vi "AO Continuous Config Pane.vi"(6 "_SubPanelMessages":refnum<notifier>, 9 "_myEmbeddedToFrameEvent":T7, 10 "_myEmbedded.Exit":refnum<user-event>, 11 "-Property Bundle":cluster{"Name":string, "Value":variant}[](array[cluster])) -> (1 "_Connection Informations":T3, 2 "_Scripter Input":T9)   [LabVIEW 2021]
doc: "Writes values to one or more analog output channels. Use this Express VI to write one or multiple samples for each channel at one time."
uses:
  <vilib>/myRIO/Common/Express VI Framework/xctls/myRIO Channel List/myRIO Channel List.xctl
  <vilib>/myRIO/Common/Express VI Framework/typedefs/Config Pane to Framework Ref.ctl
  <vilib>/myRIO/Common/Express VI Framework/typedefs/Data Validate Ref.ctl
  <vilib>/myRIO/Common/Express VI Framework/typedefs/Scripter Input.ctl
  <vilib>/myRIO/Common/Express VI Framework/typedefs/WireThrough Terminal Names.ctl
  <vilib>/myRIO/Common/Express VI Framework/typedefs/Instrument Driver Method Descriptor Array.ctl
  <vilib>/myRIO/Common/Express VI Framework/typedefs/Instrument Driver Method Descriptor.ctl
  <vilib>/myRIO/Common/Express VI Framework/typedefs/Sub Panel Messages.ctl
  <vilib>/myRIO/Common/Express VI Framework/typedefs/Connection Informations.ctl
  <vilib>/myRIO/Common/Instrument Driver Framework/Utilities/typedefs/Channel Types.ctl
  <vilib>/myRIO/Common/Express VI Framework/vis/Express VI Framework Strings Global.vi
panel:
  in  "Timeout":i32=-1 caption="Timeout:"
  in  "Sample Rate Unit":string="kHz"
  out "_learnMoreLatency":string="No gap exists during continuous generation. Learn more"
  out "_learnMoreFrequency":string="Detailed information about valid update rates for this Express VI. Learn more"
  in  "Wait Until Done?":bool caption="Wait until done?"
  in  "_Validate":bool
  in  "Sample Rate:":dbl=1.0 caption="Update rate:"
  in  "Name:":string="Analog output (continuous)" caption="Node name:"
  in  "Selected Channel List":T1[](xcontrol)=[{"Channel Name"=0, "Channel Alias"="", "Remove Channel"=FALSE, "Index"=0}]
  in  "_Default Alias String":string
  in  "_VI Default Name (Edit and make value default)":string="Analog output (continuous)"
  in  "_WireThrough Info (Edit and make value default)":T4={"WireThrough Top In"="AO (Continuous) Ref In", "WireThrough Bottom In"="error in (no error)", "WireThrough Top Out"="AO (Continuous) Ref Out", "WireThrough Bottom Out"="error out"}
  in  "_Template Array (Edit and make value default)":T5=[{"Function Name"="AO Continuous Smart Write", "VI Path"=path "<vilib>/myRIO/Instrument Drivers/Onboard IO/AO Continuous/vis", "Script"=TRUE, "Inputs"=[{"name"="Channel Names", "value"=variant, "Config Pane Only"=TRUE, "Build Array"=FALSE, "Bundle Cluster"=FALSE, "Show Term"=FALSE, "alias"=[], "Required Input"=FALSE}, {"name"="Sample Rate", "value"=variant, "Config Pane Only"=TRUE, "Build Array"=FALSE, "Bundle Cluster"=FALSE, "Show Term"=FALSE, "alias"=[], "Required Input"=FALSE}, {"name"="Data To Write", "value"=variant, "Config Pane Only"=FALSE, "Build Array"=TRUE, "Bundle Cluster"=FALSE, "Show Term"=TRUE, "alias"=[], "Required Input"=TRUE}, {"name"="Timeout", "value"=variant, "Config Pane Only"=TRUE, "Build Array"=FALSE, "Bundle Cluster"=FALSE, "Show Term"=FALSE, "alias"=[], "Required Input"=FALSE}, {"name"="Wait Until Done?", "value"=variant, "Config Pane Only"=TRUE, "Build Array"=FALSE, "Bundle Cluster"=FALSE, "Show Term"=FALSE, "alias"=[], "Required Input"=FALSE}, {"name"="Stop?", "value"=variant, "Config Pane Only"=FALSE, "Build Array"=FALSE, "Bundle Cluster"=FALSE, "Show Term"=TRUE, "alias"=[], "Required Input"=TRUE}], "Outputs"=[], "VI Class"=enum."Open", "Controls Refs[]"=[], "Inline"=TRUE}]
  in  "_Test Close":bool
  # "User Visible Area"
  # "NOTE: Tab Order has been set\nfor this Front Panel.\n1. Name: (string control)\n2. Add Channel (button)\n3. Selected Channel List (array)\n\nAll other controls are excluded \nfrom Tabbing order\n\nTo exlude a control from context\nhelp prefix its label text with a '-'"
  # "kS/s"
  # "ms"
  # "When you set Stop? terminal to TRUE, this Express VI waits until the write operation completes."
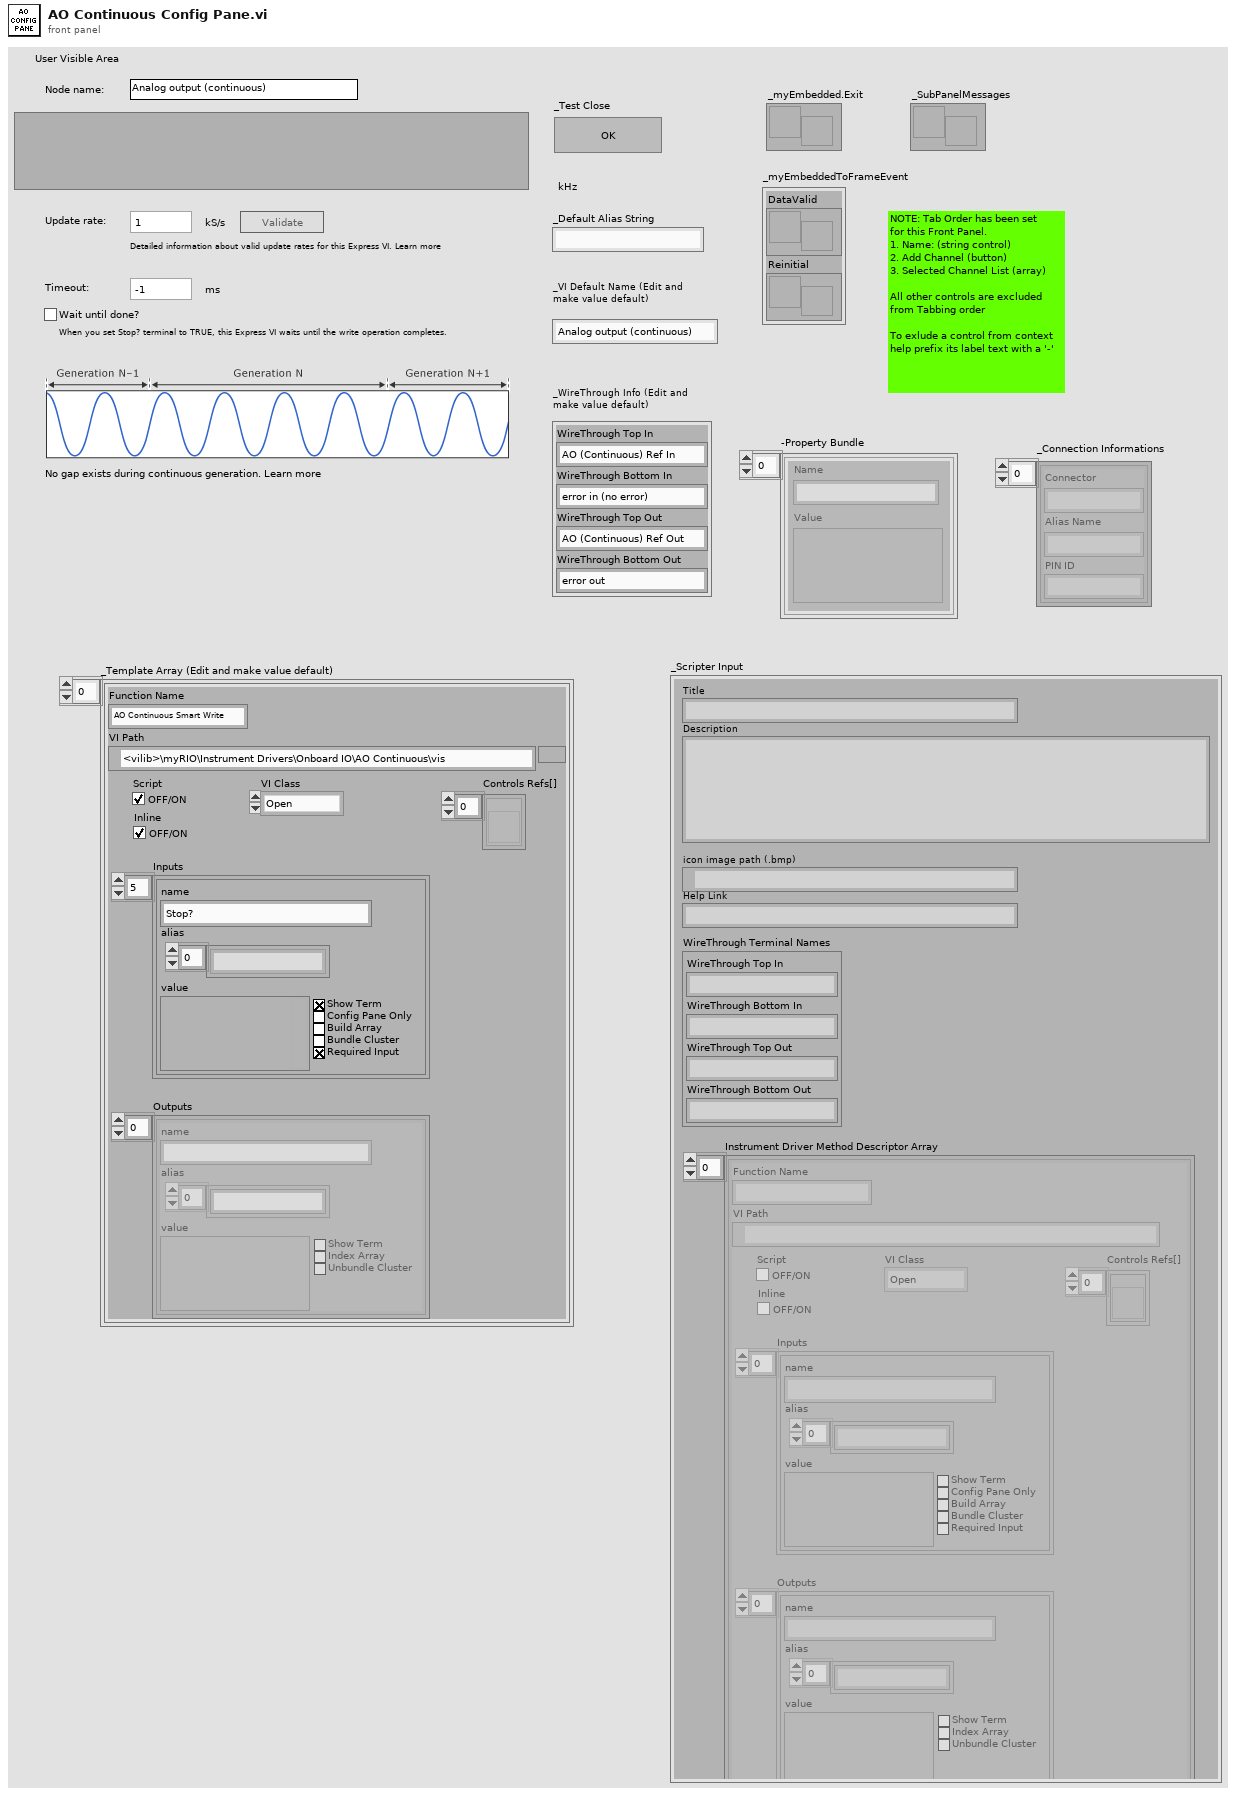
[diagram p1: front panel]
types:
  T1 = typedef "myRIO Channel List.xctl/Channel Data.ctl" = cluster{"Channel Name":u16, "Channel Alias":string, "Remove Channel":T2, "Index":i32}
  T2 = typedef "myRIO Channel List.xctl/Remove Channel.ctl" = bool
  T3 = typedef "Connection Informations.ctl" = cluster{"Connector":string, "Alias Name":string, "PIN ID":string}[]
  T4 = typedef "WireThrough Terminal Names.ctl" = cluster{"WireThrough Top In":string, "WireThrough Bottom In":string, "WireThrough Top Out":string, "WireThrough Bottom Out":string}
  T5 = typedef "Instrument Driver Method Descriptor Array.ctl" = T6[]
  T6 = typedef "Instrument Driver Method Descriptor.ctl" = cluster{"Function Name":string, "VI Path":path, "Script":bool, "Inputs":cluster{"name":string, "value":variant, "Config Pane Only":bool, "Build Array":bool, "Bundle Cluster":bool, "Show Term":bool, "alias":string[], "Required Input":bool}[], "Outputs":cluster{"name":string, "value":variant, "Show Term":bool, "Index Array":bool, "Unbundle Cluster":bool, "alias":string[]}[], "VI Class":enum16{"Open", "Configure", "Data", "Manage", "Close"}, "Controls Refs[]":refnum<vi>[], "Inline":bool}
  T7 = typedef "Config Pane to Framework Ref.ctl" = cluster{"DataValid":T8, "Reinitial":refnum<user-event>}
  T8 = typedef "Data Validate Ref.ctl" = refnum<user-event>
  T9 = typedef "Scripter Input.ctl" = cluster{"Title":string, "Description":string, "icon image path (.bmp)":path, "Help Link":string, "WireThrough Terminal Names":T4, "Instrument Driver Method Descriptor Array":T5}
  T10 = typedef "Channel Types.ctl" = enum32{"Unknown", "AI", "AO", "DIO - DI", "DIO", "DIO - DO", "I2C", "PWM", "Encoder", "SPI", "UART", "Accelerometer", "DIO - LED", "DIO - Button", "AI (N Samples)", "AudioIn (N Samples)", "AO (N Samples)", "AudioOut (N Samples)", "DI (N Samples)", "DO (N Samples)", "AI IRQ", "DI IRQ", "Timer IRQ", "RSL", "Relay", "CAN", "AI (Continuous)", "AO (Continuous)"}
  T11 = typedef "Channel Info.ctl" = cluster{"Channel Name":string, "Alias":string, "Used?":bool, "Not Support?":bool, "Property Bundle":cluster{"Name":string, "Value":variant}[]}
  T12 = typedef "Sub Panel Messages.ctl" = enum16{"Initialized"}
  T13 = enum8{"Enabled", "Disabled", "Disabled and Grayed Out"}
  T14 = cluster{"Connector":string, "Alias Name":string, "PIN ID":string}[]
  T15 = cluster{"name":string, "value":variant, "Config Pane Only":bool, "Build Array":bool, "Bundle Cluster":bool, "Show Term":bool, "alias":string[], "Required Input":bool}[]
  T16 = cluster{"name":string, "value":variant, "Config Pane Only":bool, "Build Array":bool, "Bundle Cluster":bool, "Show Term":bool, "alias":string[], "Required Input":bool}
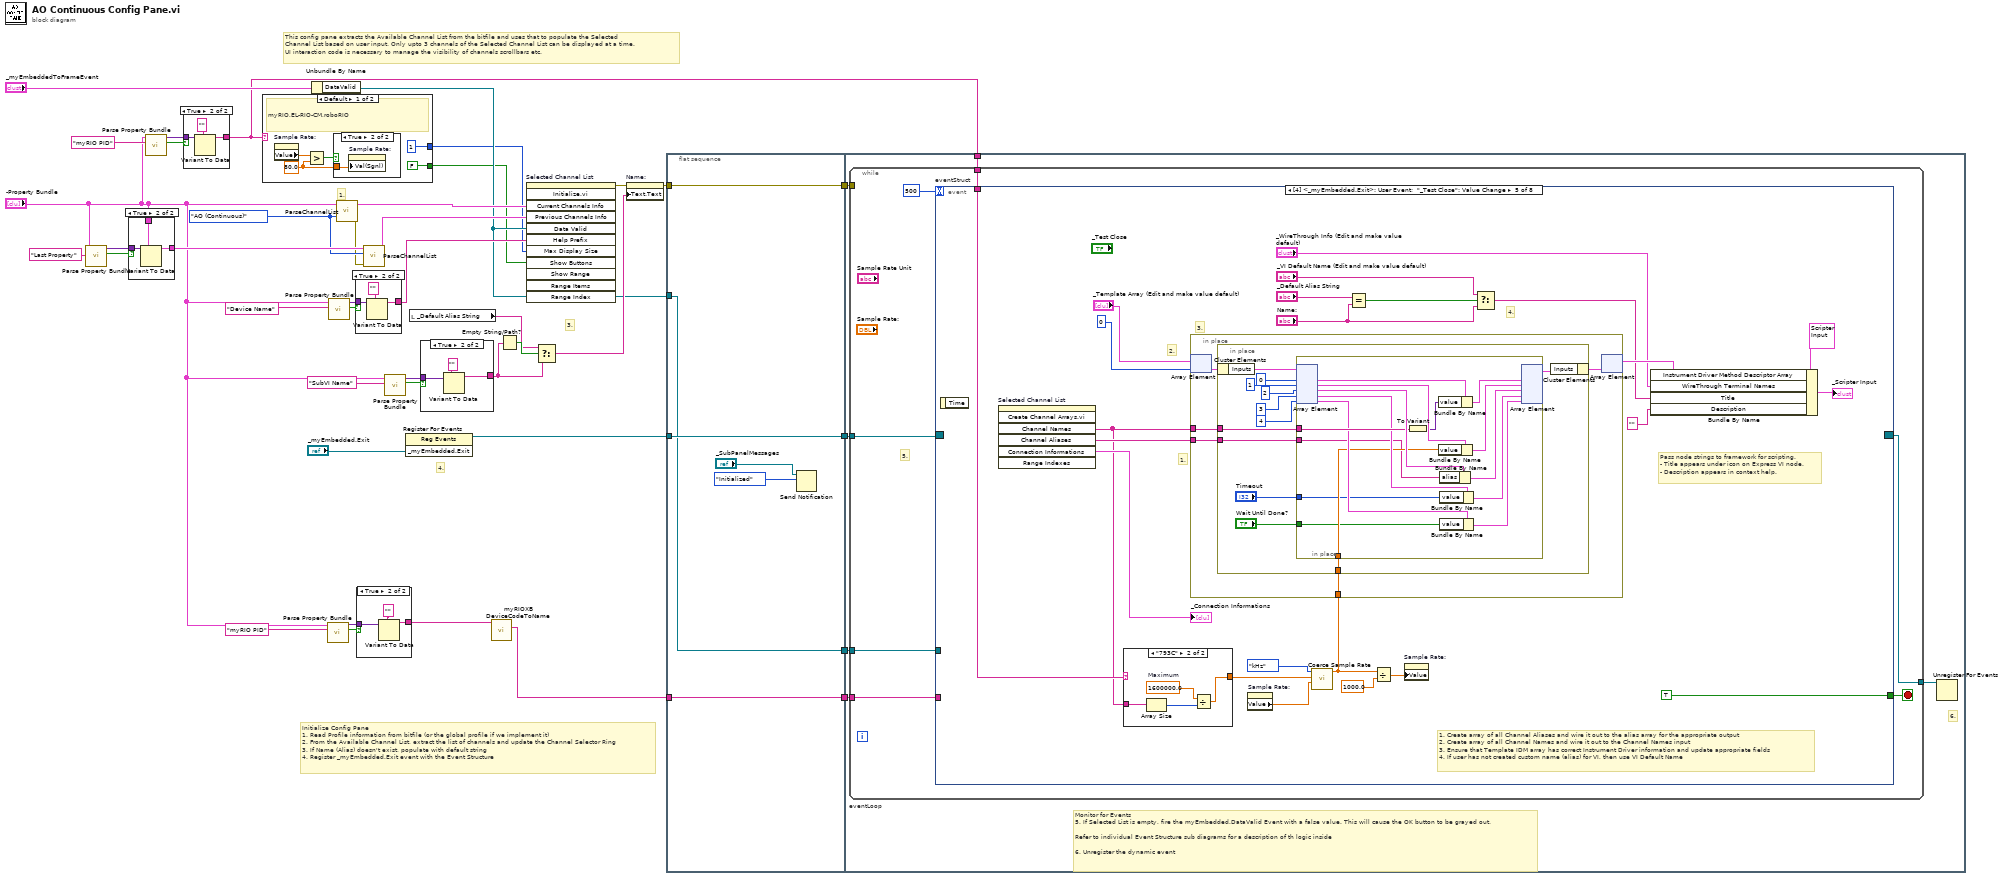
[diagram p0: block diagram]
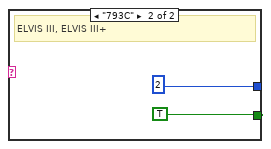
[diagram p3: hidden frame]
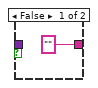
[diagram p4: hidden frame]
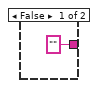
[diagram p5: hidden frame]
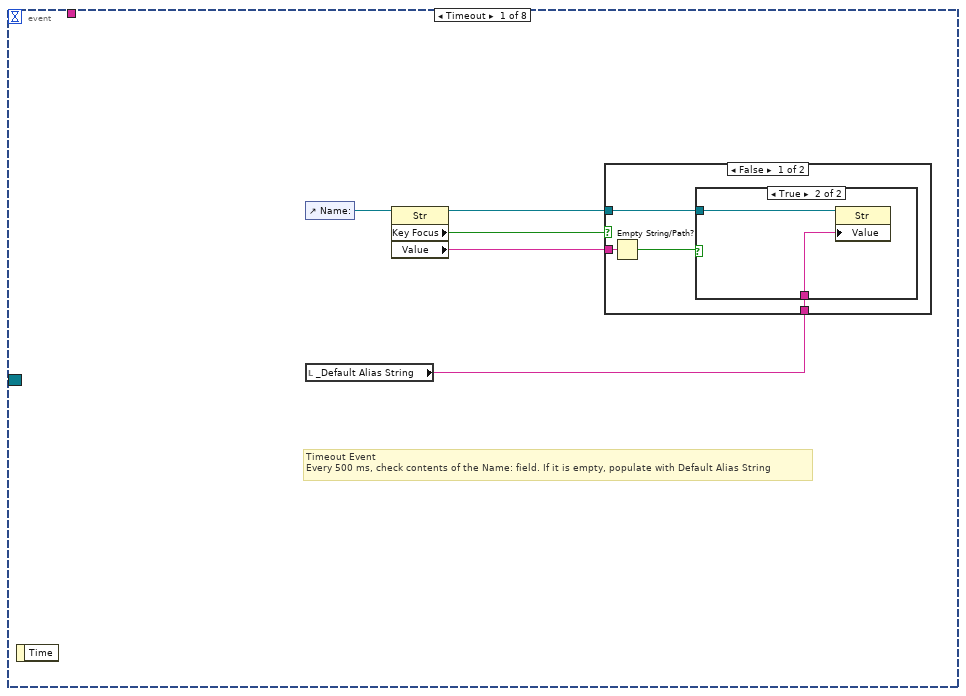
[diagram p6: hidden frame]
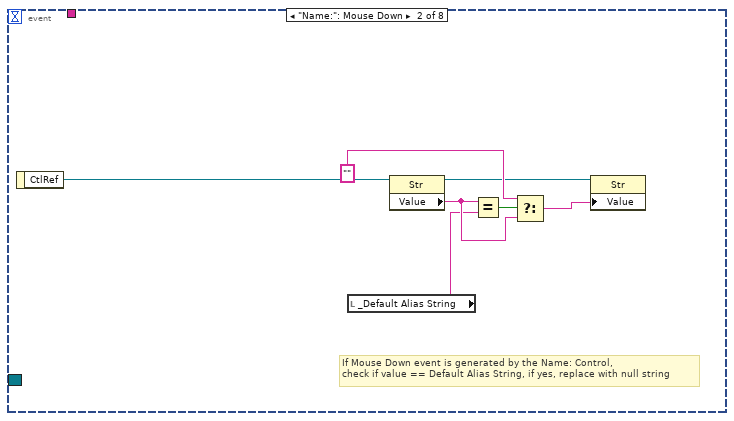
[diagram p9: hidden frame]
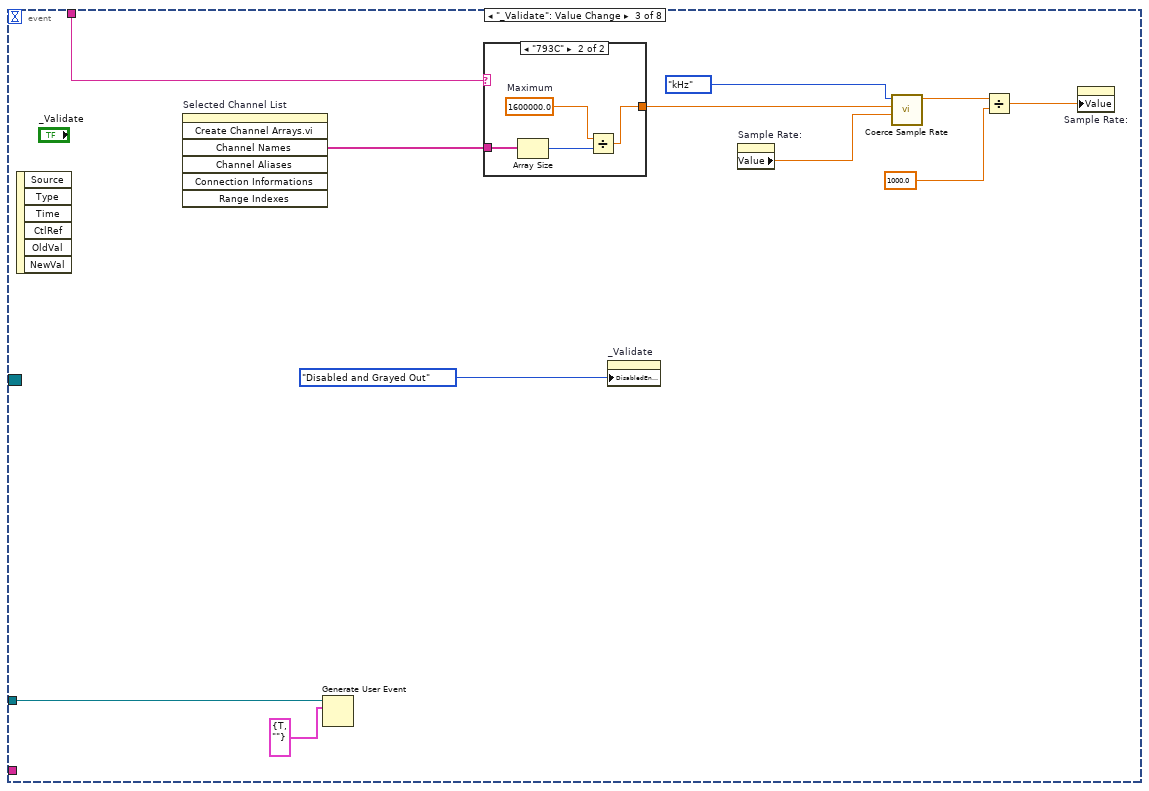
[diagram p10: hidden frame]
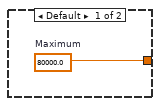
[diagram p11: hidden frame]
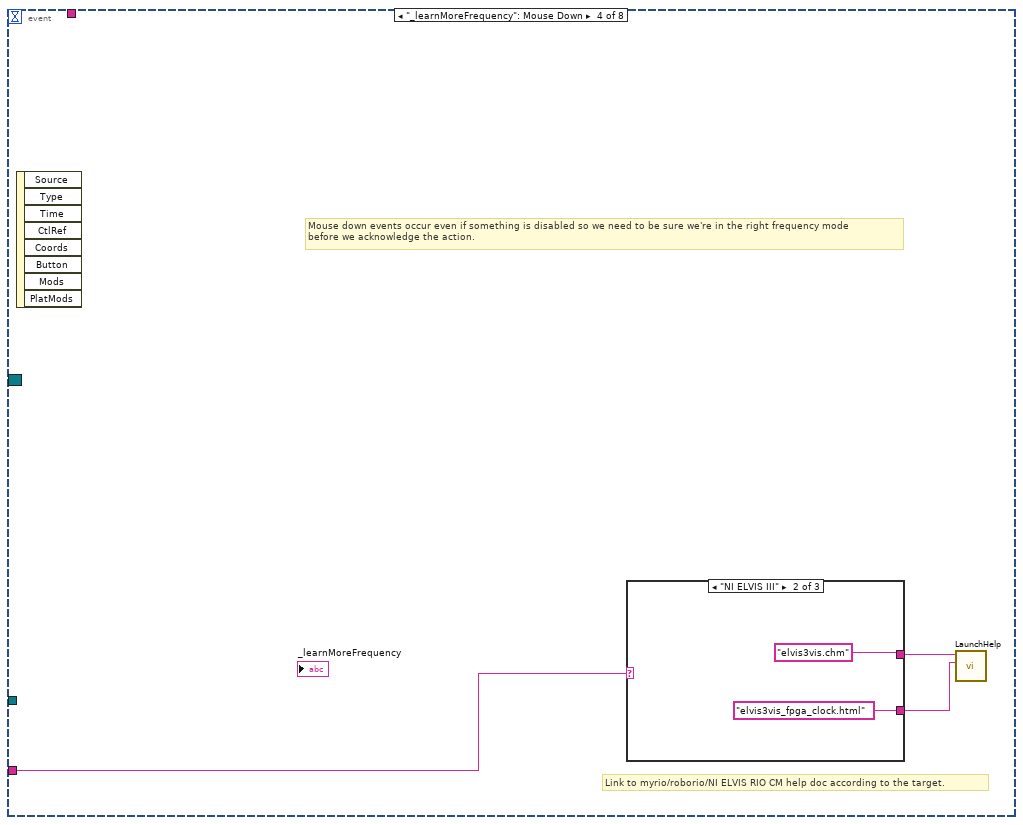
[diagram p12: hidden frame]
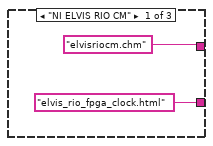
[diagram p13: hidden frame]
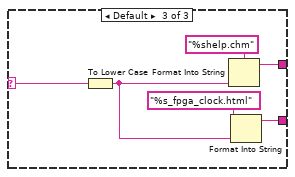
[diagram p14: hidden frame]
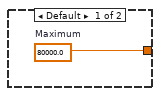
[diagram p15: hidden frame]
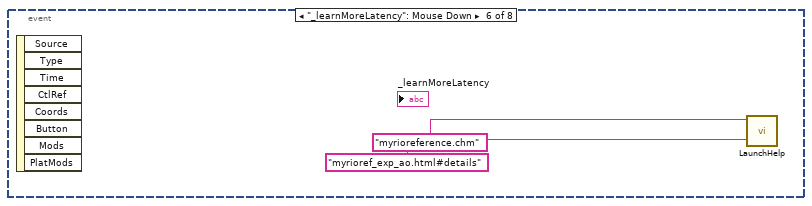
[diagram p16: hidden frame]
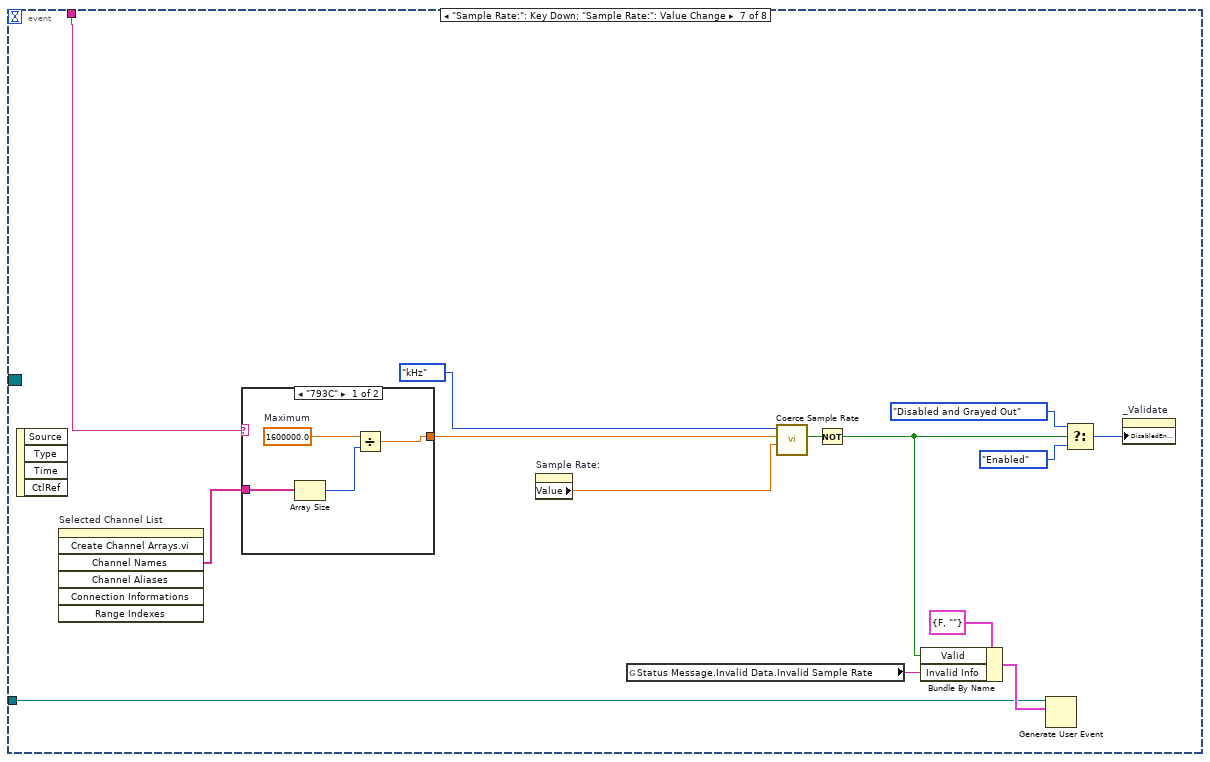
[diagram p17: hidden frame]
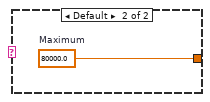
[diagram p18: hidden frame]
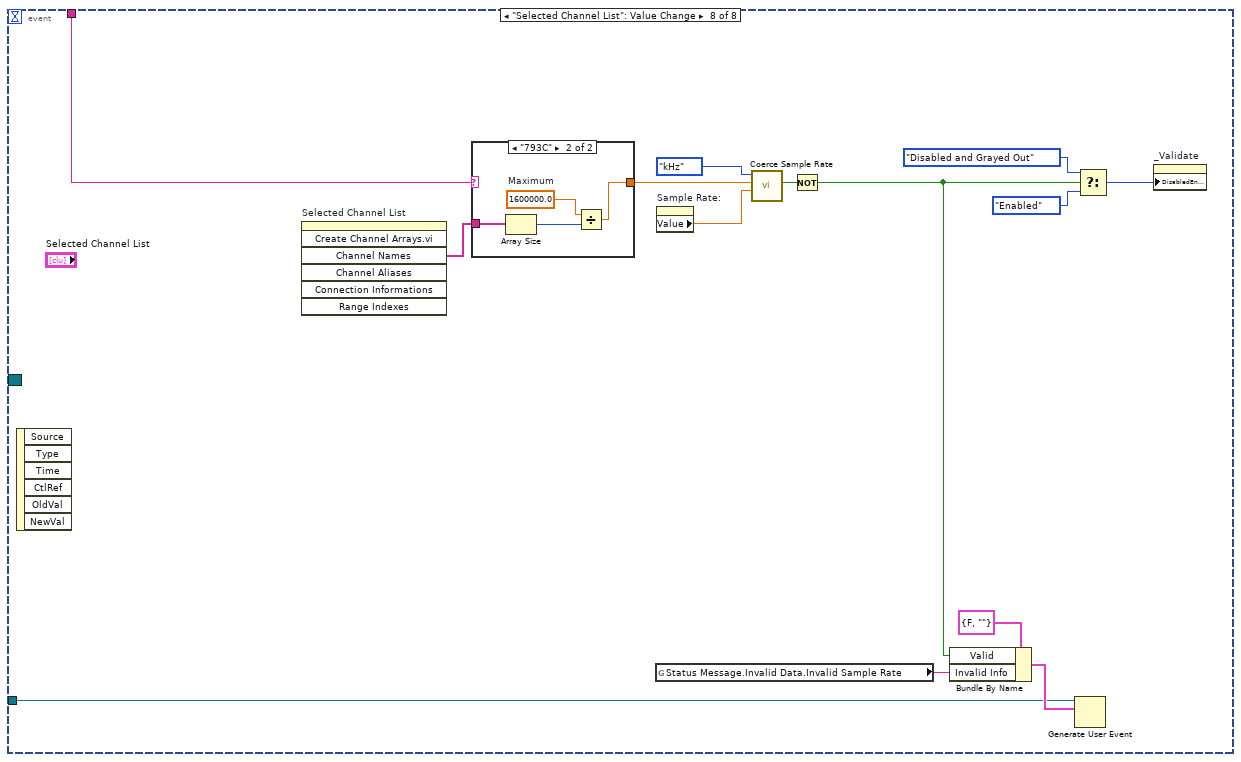
[diagram p19: hidden frame]
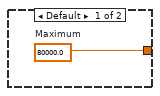
[diagram p20: hidden frame]
diagram:
  w25 = Channel_Types."AO (Continuous)" ("Channel to Read")
  # "3."
  # "1."
  # "This config pane extracts the Available Channel List from the bitfile and uses that to populate the Selected \nChannel List based on user input. Only upto 3 channels of the Selected Channel List can be displayed at a time. \nUI interaction code is necessary to manage the visibility of channels scrollbars etc."
  # "4."
  # "Initialize Config Pane\n1. Read Profile information from bitfile (or the global profile if we implement it)\n2. From the Available Channel List, extract the list of channels and update the Channel Selector Ring\n3. If Name (Alias) doesn't exist, populate with default string\n4. Register _myEmbedded.Exit event with the Event Structure"
  n1 = call <vilib>:"Parse Property Bundle.vi"("Name"="Last Property", "Property Bundle"="-Property Bundle") -> ("Found?"=w27:bool, "Value"=w28:variant)  [unwired: 8 in]
  n2 = case shown="True" w27 {
    tunnel: w28 -> [_ w44]
    tunnel: [_ w43] -> w26
    tunnel: "-Property Bundle" -> [_ w42]
    frame False {
    }
    frame True {
      n3 = Variant To Data(type=w42, Variant=w44) -> (data=w43:cluster{"Name":string, "Value":variant}[])  [unwired: 1 in, 1 out]
    }
  }
  n4 = call <vilib>:"Parse Property Bundle.vi"("Name"="myRIO PID", "Property Bundle"="-Property Bundle") -> ("Found?"=w4:bool, "Value"=w5:variant)  [unwired: 8 in]
  n5 = case shown="True" w4 {
    tunnel: w5 -> [_ w48]
    tunnel: ["" ("Name") w47] -> w1
    frame False {
    }
    frame True {
      n6 = Variant To Data(type="" ("Name"), Variant=w48) -> (data=w47:string)  [unwired: 1 in, 1 out]
    }
  }
  n7 = case shown="Default" w1 {
    tunnel: [FALSE TRUE] -> w3
    tunnel: [1 ("Max Display Size") 2 ("Max Display Size")] -> w2
    frame Default {
      w49 = 80.0 ("y")
      # "myRIO,EL-RIO-CM,roboRIO"
      n8 = property on="Sample Rate:" class="DigNum (strict)"() -> ("Value"=w51:dbl)  [unwired: 2 in, 2 out]
      n9 = Greater?(x=w51, y=w49) -> (0:w50:bool)
      n10 = case shown="True" w50 {
        tunnel: w49 -> [_ w54]
        frame False {
        }
        frame True {
          n11 = property on="Sample Rate:" class="DigNum (strict)"("Val(Sgnl)"=w54) -> ()  [unwired: 2 in, 2 out]
        }
      }
    }
    frame "793C" {
      # "ELVIS III, ELVIS III+"
    }
  }
  n12 = Unbundle By Name("_myEmbeddedToFrameEvent") -> ("DataValid"=w15:T8)
  n13 = call <vilib>:"Parse Property Bundle.vi"("Name"="myRIO PID", "Property Bundle"="-Property Bundle") -> ("Found?"=w11:bool, "Value"=w12:variant)  [unwired: 8 in]
  n14 = call <vilib>:"Parse Property Bundle.vi"("Name"="Device Name", "Property Bundle"="-Property Bundle") -> ("Found?"=w21:bool, "Value"=w20:variant)  [unwired: 8 in]
  n15 = call <vilib>:"ParseChannelList.vi"("Channel to Read"=w25, "_Property Bundle"="-Property Bundle") -> ("error out"=w23:errorcluster, "Channel List Out"=w32:T11[])  [unwired: 7 in, 1 out]
  n16 = case shown="True" w21 {
    tunnel: w20 -> [_ w59]
    tunnel: [_ w58] -> w18
    frame False {
    }
    frame True {
      n17 = Variant To Data(type="", Variant=w59) -> (data=w58:string)  [unwired: 1 in, 1 out]
    }
  }
  n18 = case shown="True" w11 {
    tunnel: w12 -> [_ w63]
    tunnel: ["" ("Name") w61] -> w9
    frame False {
    }
    frame True {
      n19 = Variant To Data(type="" ("Name"), Variant=w63) -> (data=w61:string)  [unwired: 1 in, 1 out]
    }
  }
  n20 = call <vilib>:"ParseChannelList.vi"("error in (no error)"=w23, "Channel to Read"=w25, "_Property Bundle"=w26) -> ("Channel List Out"=w24:T11[])  [unwired: 6 in, 2 out]
  n21 = call <vilib>:"Parse Property Bundle.vi"("Name"="SubVI Name", "Property Bundle"="-Property Bundle") -> ("Found?"=w35:bool, "Value"=w34:variant)  [unwired: 8 in]
  n22 = register-events("_myEmbedded.Exit") -> (reference out=w41:refnum<event-registration>)  [unwired: 2 in, 1 out]
  n23 = local read "_Default Alias String"() -> (w31:string)
  n24 = case shown="True" w35 {
    tunnel: w34 -> [_ w67]
    tunnel: ["" ("Name") w65] -> w33
    frame False {
    }
    frame True {
      n25 = Variant To Data(type="" ("Name"), Variant=w67) -> (data=w65:string)  [unwired: 1 in, 1 out]
    }
  }
  n26 = call <vilib>:"myRIOXB DeviceCodeToName.vi"("Device Code"=w9) -> ("Name"=w8:string)  [unwired: 10 in]
  n27 = Empty String/Path?(string/path=w33) -> (empty?=w39:bool)
  n28 = invoke on="Selected Channel List" class="myRIO Channel List (strict)" method="Initialize.vi"("Current Channels Info"=w32, "Previous Channels Info"=w24, "Data Valid"=w15, "Help Prefix"=w18, "Max Display Size"=w2, "Show Buttons"=w3) -> (error out=w30:errorcluster)  [unwired: 6 in, 11 out]
  n29 = Select(t=w31, s=w39, f=w33) -> (s? t:f=w38:string)
  n30 = property on="Name:" class="Str"(error in=w30, "Text.Text"=w38) -> (error out=w37:errorcluster)  [unwired: 1 in, 1 out]
  n31 = flat-sequence {
    tunnel: w37 -> [w72]
    tunnel: w41 -> [w73]
    tunnel: [w73] -> w17
    tunnel: [w72] -> w16
    tunnel: w15 -> [w69]
    tunnel: [w69] -> w14
    tunnel: [w68] -> w10
    tunnel: w8 -> [w68]
    tunnel: w17 -> [w79]
    tunnel: w16 -> [w77]
    tunnel: w14 -> [w76]
    tunnel: w10 -> [w75]
    tunnel: w1 -> [w74]
    frame #0 {
      n32 = Send Notification(notification=Sub_Panel_Messages."Initialized", notifier="_SubPanelMessages") -> ()  [unwired: 1 in, 2 out]
    }
    frame #1 {
      # "6."
      # "Monitor for Events\n5. If Selected List is empty, fire the myEmbedded.DataValid Event with a false value. This will cause the OK button to be grayed out.\n\nRefer to individual Event Structure sub diagrams for a description of th logic inside\n\n6. Unregister the dynamic event"
      n33 = while "eventLoop" {
        tunnel: w79 -> [w85]
        tunnel: [w84] -> w78
        tunnel: w77 -> [_]
        tunnel: w76 -> [w82]
        tunnel: w75 -> [w81]
        tunnel: w74 -> [w80]
        stop <- w86 stop-if-true
        # "5."
        n34 = event "eventStruct" shown="[4] <_myEmbedded.Exit>: User Event;  \"_Test Close\": Value Change" {
          selector: w85 -> [_ _ _ _ _ _ _ _]
          dyn-events: [_ _ _ _ _ _ _ _] -> w84
          timeout: 500 -> [_ _ _ _ _ _ _ _]
          tunnel: [_ _ _ _ TRUE ("_Test Close") _ _ _] -> w86
          tunnel: w82 -> [_ _ w108 _ _ _ w207 w221]
          tunnel: w81 -> [_ _ _ w121 _ _ _ _]
          tunnel: w80 -> [_ _ w107 _ w135 _ w203 w225]
          event Timeout {
            # "Timeout Event\nEvery 500 ms, check contents of the Name: field. If it is empty, populate with Default Alias String"
            n35 = event-data() -> ()  [unwired: 1 in, 1 out]
            n36 = control-ref of="Name:"() -> (w89:refnum<vi>)
            n37 = local read "_Default Alias String"() -> (w87:string)
            n38 = property on="Property Node" class="Str"(reference=w89) -> (reference out=w88:refnum<vi>, "Key Focus"=w90:bool, "Value"=w91:string)  [unwired: 1 in, 1 out]
            n39 = case shown="False" w90 {
              tunnel: w91 -> [w95 _]
              tunnel: w88 -> [w93 _]
              tunnel: w87 -> [w92 _]
              frame False {
                n40 = Empty String/Path?(string/path=w95) -> (empty?=w94:bool)
                n41 = case shown="True" w94 {
                  tunnel: w93 -> [_ w97]
                  tunnel: w92 -> [_ w96]
                  frame False {
                  }
                  frame True {
                    n42 = property on="Property Node" class="Str"(reference=w97, "Value"=w96) -> ()  [unwired: 1 in, 2 out]
                  }
                }
              }
              frame True {
              }
            }
          }
          event "Name:": Mouse Down {
            # "If Mouse Down event is generated by the Name: Control,\ncheck if value == Default Alias String, if yes, replace with null string"
            n43 = event-data() -> ("CtlRef"=w104:refnum<vi>)  [unwired: 1 in]
            n44 = local read "_Default Alias String"() -> (w98:string)
            n45 = property class="Str"(reference=w104) -> (reference out=w100:refnum<vi>, "Value"=w99:string)  [unwired: 1 in, 1 out]
            n46 = Equal?(x=w99, y=w98) -> (x = y?=w103:bool)
            n47 = Select(t="", s=w103, f=w99) -> (s? t:f=w101:string)
            n48 = property class="Str"(reference=w100, "Value"=w101) -> ()  [unwired: 1 in, 2 out]
          }
          event "_Validate": Value Change {
            n49 = event-data() -> ()  [unwired: 1 in, 6 out]
            n50 = invoke on="Selected Channel List" class="myRIO Channel List (strict)" method="Create Channel Arrays.vi"() -> ("Channel Names"=w105:string[])  [unwired: 7 in, 6 out]
            n51 = Generate User Event(user event=w108, event data cluster=cluster{"Valid":bool, "Invalid Info":string} {"Valid"=TRUE, "Invalid Info"=""} ("event data")) -> ()  [unwired: 2 in, 2 out]
            n52 = case shown="\"793C\"" w107 {
              tunnel: [w116 w119] -> w106
              tunnel: w105 -> [_ w120]
              frame Default {
                w116 = 80000.0  # Maximum
              }
              frame "793C" {
                w118 = 1600000.0  # Maximum
                n53 = Array Size(array=w120) -> (size(s)=w117:i32)
                n54 = Divide(x=w118, y=w117) -> (x/y=w119:dbl)
              }
            }
            n55 = property on="_Validate" class="Bool"("DisabledEnum"=T13."Disabled and Grayed Out" ("Disabled")) -> ()  [unwired: 2 in, 2 out]
            n56 = property on="Sample Rate:" class="DigNum (strict)"() -> ("Value"=w115:dbl)  [unwired: 2 in, 2 out]
            n57 = call <vilib>:"Coerce Sample Rate.vi"("Sample Rate:"=w115, "Maximum"=w106, "Sample Rate Unit"=enum16{"Hz", "kHz", "MHz"}."kHz") -> ("Actual Sample Rate (s)"=w112:dbl)  [unwired: 7 in, 1 out]
            n58 = Divide(x=w112, y=1000.0) -> (x/y=w110:dbl)
            n59 = property on="Sample Rate:" class="DigNum (strict)"("Value"=w110) -> ()  [unwired: 2 in, 2 out]
          }
          event "_learnMoreFrequency": Mouse Down {
            # "Link to myrio/roborio/NI ELVIS RIO CM help doc according to the target."
            # "Mouse down events occur even if something is disabled so we need to be sure we're in the right frequency mode\nbefore we acknowledge the action."
            n60 = event-data() -> ()  [unwired: 1 in, 8 out]
            n61 = case shown="\"NI ELVIS III\"" w121 {
              selector: w121 -> [_ _ w128]
              tunnel: ["elvisriocm.chm" ("Help File") "elvis3vis.chm" ("Help File") w130] -> w123
              tunnel: ["elvis_rio_fpga_clock.html" ("Help Topic") "elvis3vis_fpga_clock.html" ("Help Topic") w129] -> w122
              frame "NI ELVIS RIO CM" {
              }
              frame "NI ELVIS III" {
              }
              frame Default {
                n62 = To Lower Case(string=w128) -> (all lower case string=w132:string)
                n63 = Format Into String(format string="%shelp.chm" ("Help File"), w132) -> (resulting string=w130:string)  [unwired: 2 in, 1 out]
                n64 = Format Into String(format string="%s_fpga_clock.html" ("Help Topic"), w132) -> (resulting string=w129:string)  [unwired: 2 in, 1 out]
              }
            }
            n65 = call <vilib>:"LaunchHelp.vi"("Help Topic"=w122, "Help File"=w123) -> ()  [unwired: 10 in]
          }
          event User Event; "_Test Close": Value Change {
            # "2."
            # "1."
            # "1. Create array of all Channel Aliases and wire it out to the alias array for the appropriate output\n2. Create array of all Channel Names and wire it out to the Channel Names input\n3. Ensure that Template IDM array has correct Instrument Driver information and update appropriate fields\n4. If user has not created custom name (alias) for VI, then use VI Default Name"
            # "4."
            # "3."
            # "Pass node strings to framework for scripting.\n- Title appears under icon on Express VI node.\n- Description appears in context help."
            n66 = event-data() -> ()  [unwired: 1 in, 1 out]
            n67 = invoke on="Selected Channel List" class="myRIO Channel List (strict)" method="Create Channel Arrays.vi"() -> ("Channel Names"=w134:string[], "Channel Aliases"=w143:string[], "Connection Informations"=→"_Connection Informations":T14)  [unwired: 7 in, 4 out]
            n68 = case shown="\"793C\"" w135 {
              tunnel: [w157 w160] -> w137
              tunnel: w134 -> [_ w161]
              frame Default {
                w157 = 80000.0  # Maximum
              }
              frame "793C" {
                w159 = 1600000.0  # Maximum
                n69 = Array Size(array=w161) -> (size(s)=w158:i32)
                n70 = Divide(x=w159, y=w158) -> (x/y=w160:dbl)
              }
            }
            n71 = property on="Sample Rate:" class="DigNum (strict)"() -> ("Value"=w141:dbl)  [unwired: 2 in, 2 out]
            n72 = call <vilib>:"Coerce Sample Rate.vi"("Sample Rate:"=w141, "Maximum"=w137, "Sample Rate Unit"=enum16{"Hz", "kHz", "MHz"}."kHz") -> ("Actual Sample Rate (s)"=w136:dbl)  [unwired: 7 in, 1 out]
            n73 = in-place {
              in-place-border: w143 -> [w166]
              in-place-border: w136 -> [w165]
              in-place-border: w134 -> [w164]
              n74 = in-place-array #1("_Template Array (Edit and make value default)", 0) -> (w163:T6)
              n75 = in-place {
                in-place-border: w166 -> [w177]
                in-place-border: w165 -> [w175]
                in-place-border: w164 -> [w173]
                n76 = in-place-cluster #2(w163) -> ("Inputs"=w178:T15)
                n77 = in-place {
                  in-place-border: w177 -> [w181]
                  in-place-border: w175 -> [w182]
                  in-place-border: "Wait Until Done?" -> [w179]
                  in-place-border: w173 -> [w188]
                  in-place-border: "Timeout" -> [w180]
                  n78 = in-place-array #3(w178, 0, 1, 2, 3, 4) -> (w194:T16, w192:T16, w191:T16, w186:T16, w184:T16)
                  n79 = To Variant(anything=w188) -> (Variant=w187:variant)
                  n80 = Bundle By Name(cluster=w194, "value"=w187) -> (w193:T16)
                  n81 = Bundle By Name(cluster=w192, "value"=w182) -> (w190:T16)
                  n82 = Bundle By Name(cluster=w191, "alias"=w181) -> (w189:T16)
                  n83 = Bundle By Name(cluster=w186, "value"=w180) -> (w185:T16)
                  n84 = Bundle By Name(cluster=w184, "value"=w179) -> (w183:T16)
                  n85 = in-place-array #3(w193, w190, w189, w185, w183) -> (w176:T15)  [unwired: 5 out]
                }
                n86 = in-place-cluster #2("Inputs"=w176) -> (w162:T6)
              }
              n87 = in-place-array #1(w162) -> (w155:T5)  [unwired: 1 out]
            }
            n88 = Equal?(x="_Default Alias String", y="Name:") -> (x = y?=w147:bool)
            n89 = Divide(x=w136, y=1000.0) -> (x/y=w138:dbl)
            n90 = property on="Sample Rate:" class="DigNum (strict)"("Value"=w138) -> ()  [unwired: 2 in, 2 out]
            n91 = Select(t="_VI Default Name (Edit and make value default)", s=w147, f="Name:") -> (s? t:f=w145:string)
            n92 = Bundle By Name(cluster=T9 {"Title"="", "Description"="", "icon image path (.bmp)"=path "", "Help Link"="", "WireThrough Terminal Names"={"WireThrough Top In"="", "WireThrough Bottom In"="", "WireThrough Top Out"="", "WireThrough Bottom Out"=""}, "Instrument Driver Method Descriptor Array"=[]} ("Scripter Input"), "Instrument Driver Method Descriptor Array"=w155, "WireThrough Terminal Names"="_WireThrough Info (Edit and make value default)", "Title"=w145, "Description"="" ("Title")) -> (→"_Scripter Input":T9)
          }
          event "_learnMoreLatency": Mouse Down {
            n93 = event-data() -> ()  [unwired: 1 in, 8 out]
            n94 = call <vilib>:"LaunchHelp.vi"("Help Topic"="myrioref_exp_ao.html#details", "Help File"="myrioreference.chm") -> ()  [unwired: 10 in]
          }
          event "Sample Rate:": Key Down; "Sample Rate:": Value Change {
            n95 = event-data() -> ()  [unwired: 1 in, 4 out]
            n96 = invoke on="Selected Channel List" class="myRIO Channel List (strict)" method="Create Channel Arrays.vi"() -> ("Channel Names"=w201:string[])  [unwired: 7 in, 6 out]
            n97 = case shown="\"793C\"" w203 {
              tunnel: [w211 w215] -> w202
              tunnel: w201 -> [w214 _]
              frame "793C" {
                w213 = 1600000.0  # Maximum
                n98 = Array Size(array=w214) -> (size(s)=w212:i32)
                n99 = Divide(x=w213, y=w212) -> (x/y=w211:dbl)
              }
              frame Default {
                w215 = 80000.0  # Maximum
              }
            }
            n100 = property on="Sample Rate:" class="DigNum (strict)"() -> ("Value"=w206:dbl)  [unwired: 2 in, 2 out]
            n101 = global read "Express VI Framework Strings Global.vi" "Status Message.Invalid Data.Invalid Sample Rate"() -> (w208:string)
            n102 = call <vilib>:"Coerce Sample Rate.vi"("Sample Rate:"=w206, "Maximum"=w202, "Sample Rate Unit"=enum16{"Hz", "kHz", "MHz"}."kHz") -> ("Coercion needed?"=w204:bool)  [unwired: 7 in, 1 out]
            n103 = Not(x=w204) -> (.not. x?=w198:bool)
            n104 = Bundle By Name(cluster=cluster{"Valid":bool, "Invalid Info":string} {"Valid"=FALSE, "Invalid Info"=""} ("event data"), "Valid"=w198, "Invalid Info"=w208) -> (w209:cluster{"Valid":bool, "Invalid Info":string})
            n105 = Generate User Event(user event=w207, event data cluster=w209) -> ()  [unwired: 2 in, 2 out]
            n106 = Select(t=T13."Disabled and Grayed Out" ("Disabled"), s=w198, f=T13."Enabled" ("Disabled")) -> (s? t:f=w197:T13)
            n107 = property on="_Validate" class="Bool"("DisabledEnum"=w197) -> ()  [unwired: 2 in, 2 out]
          }
          event "Selected Channel List": Value Change {
            n108 = event-data() -> ()  [unwired: 1 in, 6 out]
            n109 = invoke on="Selected Channel List" class="myRIO Channel List (strict)" method="Create Channel Arrays.vi"() -> ("Channel Names"=w227:string[])  [unwired: 7 in, 6 out]
            n110 = case shown="\"793C\"" w225 {
              tunnel: [w230 w233] -> w228
              tunnel: w227 -> [_ w234]
              frame Default {
                w230 = 80000.0  # Maximum
              }
              frame "793C" {
                w232 = 1600000.0  # Maximum
                n111 = Array Size(array=w234) -> (size(s)=w231:i32)
                n112 = Divide(x=w232, y=w231) -> (x/y=w233:dbl)
              }
            }
            n113 = global read "Express VI Framework Strings Global.vi" "Status Message.Invalid Data.Invalid Sample Rate"() -> (w222:string)
            n114 = property on="Sample Rate:" class="DigNum (strict)"() -> ("Value"=w229:dbl)  [unwired: 2 in, 2 out]
            n115 = call <vilib>:"Coerce Sample Rate.vi"("Sample Rate:"=w229, "Maximum"=w228, "Sample Rate Unit"=enum16{"Hz", "kHz", "MHz"}."kHz") -> ("Coercion needed?"=w220:bool)  [unwired: 7 in, 1 out]
            n116 = Not(x=w220) -> (.not. x?=w219:bool)
            n117 = Bundle By Name(cluster=cluster{"Valid":bool, "Invalid Info":string} {"Valid"=FALSE, "Invalid Info"=""} ("event data"), "Valid"=w219, "Invalid Info"=w222) -> (w223:cluster{"Valid":bool, "Invalid Info":string})
            n118 = Generate User Event(user event=w221, event data cluster=w223) -> ()  [unwired: 2 in, 2 out]
            n119 = Select(t=T13."Disabled and Grayed Out" ("Disabled"), s=w219, f=T13."Enabled" ("Disabled")) -> (s? t:f=w218:T13)
            n120 = property on="_Validate" class="Bool"("DisabledEnum"=w218) -> ()  [unwired: 2 in, 2 out]
          }
        }
      }
      n121 = Unregister For Events(event registration refnum=w78) -> ()  [unwired: 1 in, 1 out]
    }
  }
